vi "broadcastReg-Test.vi"() -> ()   [LabVIEW 2017]
panel:
  out "Pass?":bool=TRUE
  in  "Array":T1(array[cluster])=[{"status"="status@source >> api@target -><register>\n", "Response Message Info"=["api"], TRUE, "Response Message Info 2"=["api"]}, {"status"="status@* >> api@target -><register>", "Response Message Info"=["api"], TRUE, "Response Message Info 2"=["api"]}, {"status"="status@source >> api@target -><register>\nstatus@source >> api2@target -><register>\nstatus@source >> api@target -><unregister>", "Response Message Info"=["api2"], TRUE, "Response Message Info 2"=["api2"]}, {"status"="status@source >> api@target -><register>\nstatus@source >> api2@target -><register>\nstatus@source >> api3@target -><register>\n", "Response Message Info"=["api", "api2", "api3"], TRUE, "Response Message Info 2"=["api", "api2", "api3"]}, {"status"="status@* >> api@target -><register>\nstatus@source >> api2@target -><register>", "Response Message Info"=["api2", "api"], TRUE, "Response Message Info 2"=["api2", "api"]}, {"status"="status@* >> api@target -><register>\nstatus@source >> api@target -><unregister>", "Response Message Info"=[], TRUE, "Response Message Info 2"=[]}, {"status"="status@source >> api@target -><register>\nstatus@source >> api2@target -><register>\nstatus@source >> api@target2 -><register>", "Response Message Info"=["api", "api2"], TRUE, "Response Message Info 2"=["api", "api2"]}, {"status"="status@* >> api@target -><register>\nstatus@source >> api@target -><register>", "Response Message Info"=["api"], TRUE, "Response Message Info 2"=["api"]}, {"status"="status@* >> api@target -><register>\nstatus@source >> api@target -><register>\nstatus@* >> api@target -><unregister>", "Response Message Info"=[], TRUE, "Response Message Info 2"=[]}, {"status"="status@source >> api@target2 -><register>\nstatus@source >> api2@target2 -><register>\nstatus@source >> api@target -><register>", "Response Message Info"=["api"], TRUE, "Response Message Info 2"=["api"]}, {"status"="status@source >> api@target2 -><register>\nstatus@source >> api2@target2 -><register>\nstatus@source >> api1@target -><register>\nstatus@source >> api2@target -><register>", "Response Message Info"=["api1", "api2"], TRUE, "Response Message Info 2"=["api1", "api2"]}, {"status"="status@source >> api@target2 -><register>\nstatus@source >> api2@target2 -><register>\nstatus@source >> api1@target -><register>\nstatus@source >> api2@target -><register>\nstatus@source >> api1@target -><unregister>", "Response Message Info"=["api2"], TRUE, "Response Message Info 2"=["api2"]}, {"status"="status@source >> api@target2 -><register>\nstatus@source >> api2@target2 -><register>\nstatus@source >> api1@target -><register>\nstatus@source >> api2@target -><register>\nstatus@source >> api2@target -><unregister>", "Response Message Info"=["api1"], TRUE, "Response Message Info 2"=["api1"]}, {"status"="status@source >> api@target2 -><register>\nstatus@source >> api2@target2 -><register>\nstatus@source >> api1@target -><register>\nstatus@source >> api2@target -><register>\nstatus@* >> api2@target -><unregister>", "Response Message Info"=["api1"], TRUE, "Response Message Info 2"=["api1"]}, {"status"="status@source >> api1@target -><register>\nstatus@source >> api2@target -><register>\nstatus@* >> api2@target -><unregister>", "Response Message Info"=["api1"], TRUE, "Response Message Info 2"=["api1"]}, {"status"="status@source >> api@target2 -><register>\nstatus@source2 >> api2@target2 -><register>\nstatus@source >> api1@target -><register>\nstatus@source2 >> api1@target -><register>\nstatus@* >> api1@target -><unregister>", "Response Message Info"=[], TRUE, "Response Message Info 2"=[]}, {"status"="status@source >> api@target2 -><register>\nstatus@source2 >> api2@target2 -><register>\nstatus@source >> api1@target -><register>\nstatus@source2 >> api1@target -><register>\nstatus@source2 >> api1@target -><unregister>", "Response Message Info"=["api1"], FALSE, "Response Message Info 2"=["api"]}]
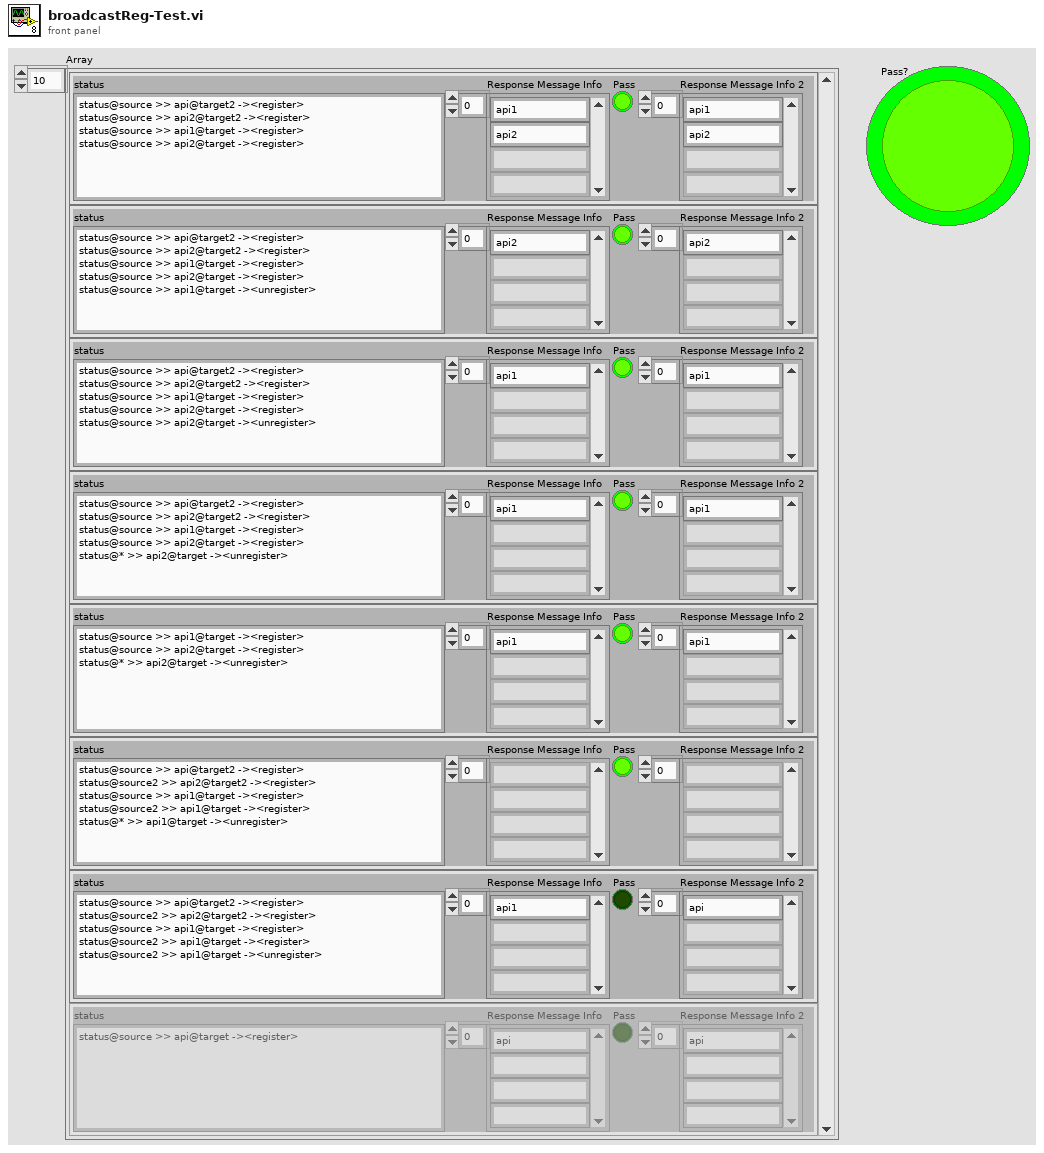
[diagram p1: front panel]
types:
  T1 = cluster{"status":string, "Response Message Info":string[], bool, "Response Message Info 2":string[]}[]
  T2 = cluster{"status":string, "Response Message Info":string[], bool, "Response Message Info 2":string[]}
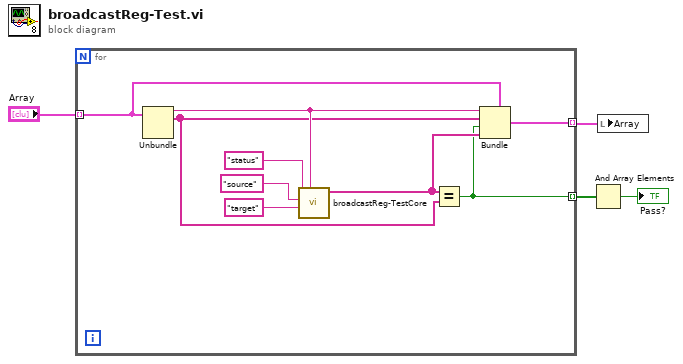
[diagram p0: block diagram]
diagram:
  n1 = for {
    tunnel: "Array" -> [w8] mode=indexing
    tunnel: [w9] -> w3 mode=indexing
    tunnel: [w5] -> w2 mode=indexing
    n2 = Unbundle(w8) -> ("status"=w10:string, "Response Message Info"=w7:string[])  [unwired: 2 out]
    n3 = call "broadcastReg-TestCore.vi"("status"=w10, "Target"="target", "Source"="source", "Status"="status") -> ("Response Message Info"=w6:string[])  [unwired: 7 in]
    n4 = Equal?(x=w6, y=w7) -> (x = y?=w5:bool)
    n5 = Bundle(cluster=w8, "status"=w10, "Response Message Info"=w7, w5, "Response Message Info 2"=w6) -> (w9:T2)
  }
  n6 = And Array Elements(Boolean array=w2) -> (logical AND=→"Pass?":bool)
  n7 = local write "Array"(w3) -> ()
